vi "Monitor Lifeline.vi"(11 "DebuggingTerminal in":refnum<class "DebuggingTerminal.lvclass">) -> (3 "Kill Process":bool)   [LabVIEW 2013, in "MQTT Base.lvlib" / "DebuggingTerminal.lvclass"]
uses:
  DebuggingTerminal.lvclass
  DebuggingTerminal.lvclass/DebuggingTerminal.ctl
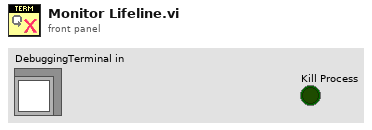
[diagram p1: front panel]
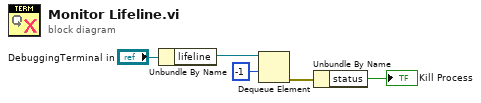
[diagram p0: block diagram]
diagram:
  n1 = Unbundle By Name("DebuggingTerminal in") -> ("lifeline"=w4:refnum<queue>)
  n2 = Dequeue Element(queue=w4, timeout in ms (-1)=-1) -> (error out=w2:errorcluster)  [unwired: 1 in, 3 out]
  n3 = Unbundle By Name(w2) -> ("status"=→"Kill Process":bool)
